vi "Croce.vi"(6 "Solo toll Y positiva?":bool=TRUE, 8 "TOLL Y %":dbl, 9 "TOLL X %":dbl, 10 "Grandezza Y":dbl, 11 "grandezza X":dbl) -> (3 "element":cluster{"X":dbl[], "Y":dbl[]})   [LabVIEW 2019]
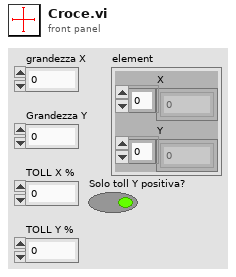
[diagram p1: front panel]
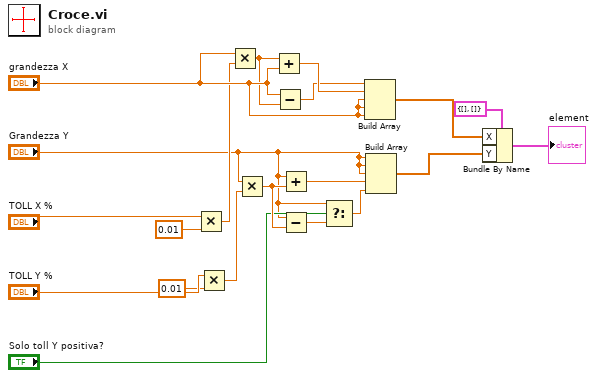
[diagram p0: block diagram]
diagram:
  n1 = Multiply(x="TOLL X %", y=0.01) -> (x*y=w10:dbl)
  n2 = Multiply(x="TOLL Y %", y=0.01) -> (x*y=w16:dbl)
  n3 = Multiply(x="grandezza X", y=w10) -> (x*y=w11:dbl)
  n4 = Multiply(x="Grandezza Y", y=w16) -> (x*y=w19:dbl)
  n5 = Add(x=w11, y="grandezza X") -> (x+y=w13:dbl)
  n6 = Subtract(x="grandezza X", y=w11) -> (x-y=w12:dbl)
  n7 = Add(x="Grandezza Y", y=w19) -> (x+y=w17:dbl)
  n8 = Subtract(x="Grandezza Y", y=w19) -> (x-y=w3:dbl)
  n9 = Select(t="Grandezza Y", s="Solo toll Y positiva?", f=w3) -> (s? t:f=w1:dbl)
  n10 = Build Array(w12, w13, "grandezza X", "grandezza X", "grandezza X") -> (w6:dbl[])
  n11 = Build Array("Grandezza Y", "Grandezza Y", "Grandezza Y", w17, w1) -> (w7:dbl[])
  n12 = Bundle By Name(cluster=cluster{"X":dbl[], "Y":dbl[]} {"X"=[], "Y"=[]} ("element"), "X"=w6, "Y"=w7) -> (→"element":cluster{"X":dbl[], "Y":dbl[]})
